vi "PSK.vi"() -> ()   [LabVIEW 2015]
panel:
  out "Waveform Graph":dbl[](graph)=[0.0, 0.9510565162951535, 0.5877852522924732, -0.5877852522924734, -0.9510565162951536, -2.4492935982947064e-16, 0.9510565162951538, 0.5877852522924734, -0.5877852522924728, -0.9510565162951538, -4.898587196589413e-16, 0.951056516295154, 0.5877852522924721, -0.5877852522924726, -0.9510565162951538, -7.347880794884119e-16, 0.9510565162951533, 0.5877852522924709, -0.5877852522924724, -0.9510565162951539, -9.797174393178826e-16, 0.9510565162951533, 0.5877852522924711, -0.5877852522924751, -0.9510565162951529, -1.2246467991473533e-15, -0.9510565162951532, -0.5877852522924742, 0.587785252292472, 0.9510565162951519, 1.4695761589768238e-15, -0.9510565162951531, -0.5877852522924744, 0.5877852522924718, 0.9510565162951519, 1.7145055188062944e-15, -0.951056516295153, -0.5877852522924746, 0.5877852522924716, 0.951056516295152, 1.959434878635765e-15, -0.9510565162951552, -0.5877852522924748, 0.5877852522924714, 0.9510565162951521, 2.204364238465236e-15, -0.9510565162951551, -0.587785252292475, 0.587785252292477, 0.9510565162951521, 2.4492935982947065e-15, 0.951056516295155, 0.5877852522924751, -0.5877852522924768, -0.9510565162951544, -9.799650315725178e-15, 0.9510565162951528, 0.5877852522924696, -0.5877852522924824, -0.9510565162951523, -2.9391523179536475e-15, 0.9510565162951549, 0.5877852522924756, -0.5877852522924764, -0.9510565162951545, 3.921345679817883e-15, 0.9510565162951525, 0.58778525229247, -0.5877852522924819, -0.9510565162951524, -3.429011037612589e-15, 0.9510565162951546, 0.587785252292476, -0.587785252292476, -0.9510565162951546, -1.0779367755043061e-14, -0.9510565162951524, -0.5877852522924705, 0.5877852522924816, 0.9510565162951525, 3.91886975727153e-15, -0.9510565162951502, -0.5877852522924649, 0.5877852522924756, 0.9510565162951549, -2.941628240500001e-15, -0.9510565162951523, -0.5877852522924708, 0.5877852522924811, 0.9510565162951528, 4.408728476930472e-15, -0.95105651629515, -0.5877852522924653, 0.5877852522924751, 0.951056516295155, 1.1759085194360944e-14, -0.9510565162951565, -0.5877852522924712, 0.5877852522924807, 0.9510565162951529, 4.898587196589413e-15, 0.9510565162951586, 0.5877852522924657, -0.5877852522924862, -0.9510565162951552, 1.9619108011821185e-15, 0.9510565162951563, 0.5877852522924601, -0.5877852522924688, -0.951056516295153, -1.9599300631450357e-14, 0.9510565162951585, 0.5877852522924776, -0.5877852522924744, -0.9510565162951509, -1.2738802633678827e-14, 0.9510565162951606, 0.587785252292472, -0.5877852522924799, -0.9510565162951575]
  out "Modulating wave 2":dbl[](graph)=[0.0, 0.9510565162951535, 0.5877852522924732, -0.5877852522924734, -0.9510565162951536, -2.4492935982947064e-16, 0.9510565162951538, 0.5877852522924734, -0.5877852522924728, -0.9510565162951538, -4.898587196589413e-16, 0.951056516295154, 0.5877852522924721, -0.5877852522924726, -0.9510565162951538, -7.347880794884119e-16, 0.9510565162951533, 0.5877852522924709, -0.5877852522924724, -0.9510565162951539, -9.797174393178826e-16, 0.9510565162951533, 0.5877852522924711, -0.5877852522924751, -0.9510565162951529, -1.2246467991473533e-15, 0.9510565162951532, 0.5877852522924742, -0.587785252292472, -0.9510565162951519, -1.4695761589768238e-15, 0.9510565162951531, 0.5877852522924744, -0.5877852522924718, -0.9510565162951519, -1.7145055188062944e-15, 0.951056516295153, 0.5877852522924746, -0.5877852522924716, -0.951056516295152, -1.959434878635765e-15, 0.9510565162951552, 0.5877852522924748, -0.5877852522924714, -0.9510565162951521, -2.204364238465236e-15, 0.9510565162951551, 0.587785252292475, -0.587785252292477, -0.9510565162951521, -2.4492935982947065e-15, 0.951056516295155, 0.5877852522924751, -0.5877852522924768, -0.9510565162951544, -9.799650315725178e-15, 0.9510565162951528, 0.5877852522924696, -0.5877852522924824, -0.9510565162951523, -2.9391523179536475e-15, 0.9510565162951549, 0.5877852522924756, -0.5877852522924764, -0.9510565162951545, 3.921345679817883e-15, 0.9510565162951525, 0.58778525229247, -0.5877852522924819, -0.9510565162951524, -3.429011037612589e-15, 0.9510565162951546, 0.587785252292476, -0.587785252292476, -0.9510565162951546, -1.0779367755043061e-14, 0.9510565162951524, 0.5877852522924705, -0.5877852522924816, -0.9510565162951525, -3.91886975727153e-15, 0.9510565162951502, 0.5877852522924649, -0.5877852522924756, -0.9510565162951549, 2.941628240500001e-15, 0.9510565162951523, 0.5877852522924708, -0.5877852522924811, -0.9510565162951528, -4.408728476930472e-15, 0.95105651629515, 0.5877852522924653, -0.5877852522924751, -0.951056516295155, -1.1759085194360944e-14, 0.9510565162951565, 0.5877852522924712, -0.5877852522924807, -0.9510565162951529, -4.898587196589413e-15, 0.9510565162951586, 0.5877852522924657, -0.5877852522924862, -0.9510565162951552, 1.9619108011821185e-15, 0.9510565162951563, 0.5877852522924601, -0.5877852522924688, -0.951056516295153, -1.9599300631450357e-14, 0.9510565162951585, 0.5877852522924776, -0.5877852522924744, -0.9510565162951509, -1.2738802633678827e-14, 0.9510565162951606, 0.587785252292472, -0.5877852522924799, -0.9510565162951575]
  out "Numeric 2":dbl=-3.4932993997482953e-16
  in  "phase 2":dbl
  in  "Amplitude 2":dbl=1.0
  in  "Fs 2":dbl=500.0
  in  "Frequency 2":dbl=100.0
  in  "No of Iteration 2":i32=120
  out "Modulating wave":dbl[](graph)=[0.0, 1.0, 1.0, 1.0, 1.0, 1.0, 1.0, 1.0, 1.0, 1.0, 1.0, 1.0, 1.0, 1.0, 1.0, 1.0, 1.0, 1.0, 1.0, 1.0, 1.0, 1.0, 1.0, 1.0, 1.0, 1.0, -1.0, -1.0, -1.0, -1.0, -1.0, -1.0, -1.0, -1.0, -1.0, -1.0, -1.0, -1.0, -1.0, -1.0, -1.0, -1.0, -1.0, -1.0, -1.0, -1.0, -1.0, -1.0, -1.0, -1.0, -1.0, 1.0, 1.0, 1.0, 1.0, 1.0, 1.0, 1.0, 1.0, 1.0, 1.0, 1.0, 1.0, 1.0, 1.0, 1.0, 1.0, 1.0, 1.0, 1.0, 1.0, 1.0, 1.0, 1.0, 1.0, 1.0, -1.0, -1.0, -1.0, -1.0, -1.0, -1.0, -1.0, -1.0, -1.0, -1.0, -1.0, -1.0, -1.0, -1.0, -1.0, -1.0, -1.0, -1.0, -1.0, -1.0, -1.0, -1.0, -1.0, -1.0, -1.0, 1.0, 1.0, 1.0, 1.0, 1.0, 1.0, 1.0, 1.0, 1.0, 1.0, 1.0, 1.0, 1.0, 1.0, 1.0, 1.0, 1.0, 1.0, 1.0]
  out "Numeric":dbl=0.014082858244057282
  in  "phase":dbl
  in  "Amplitude":dbl=1.0
  in  "Fs":dbl=1000.0
  in  "Frequency":dbl=20.0
  in  "No of Iteration":i32=120
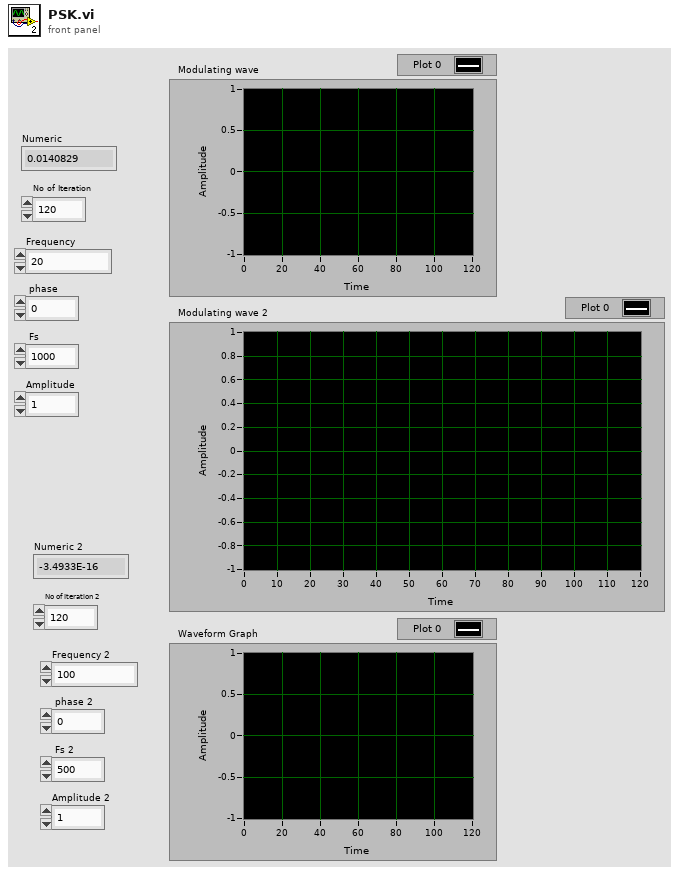
[diagram p1: front panel]
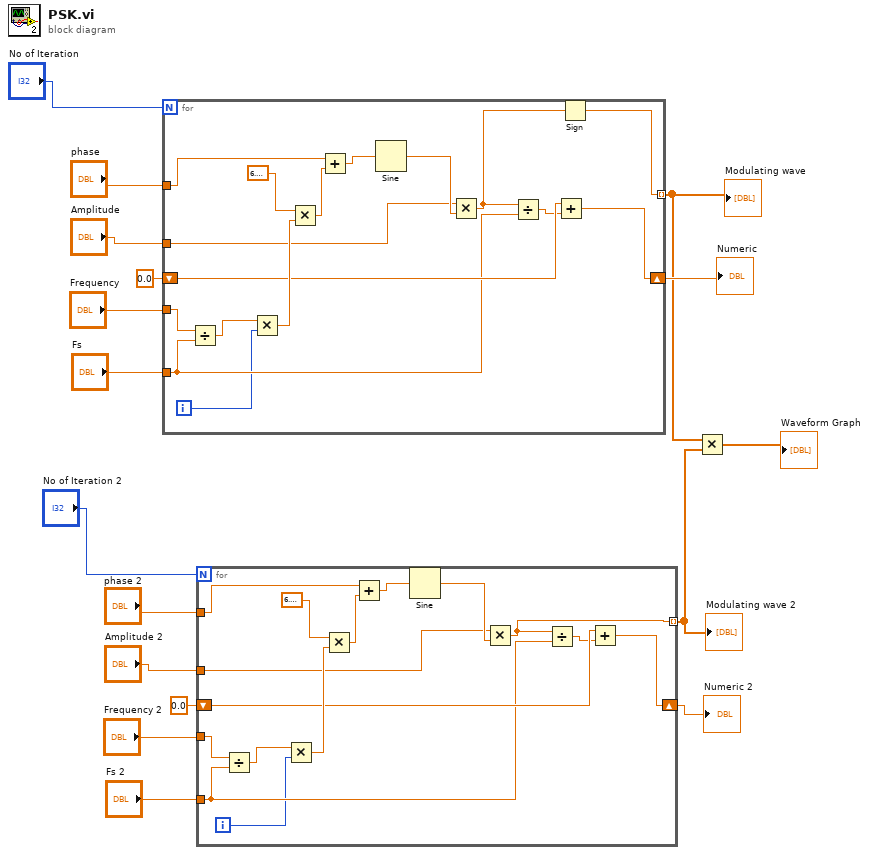
[diagram p0: block diagram]
diagram:
  n1 = for {
    N: "No of Iteration" -> [_]
    tunnel: "Frequency" -> [w32]
    tunnel: "Fs" -> [w22]
    tunnel: "Amplitude" -> [w28]
    tunnel: "phase" -> [w27]
    shift-right: [w20] -> w12
    shift-left: 0.0 -> [w25]
    tunnel: [w19] -> w2 mode=indexing
    i -> [w21]
    n2 = Divide(x=w32, y=w22) -> (x/y=w26:dbl)
    n3 = Multiply(x=w26, y=w21) -> (x*y=w30:dbl)
    n4 = Multiply(x=6.283185307179586, y=w30) -> (x*y=w31:dbl)
    n5 = Add(x=w27, y=w31) -> (x+y=w33:dbl)
    n6 = Sine(x=w33) -> (sin(x)=w29:dbl)
    n7 = Multiply(x=w28, y=w29) -> (x*y=w18:dbl)
    n8 = Divide(x=w18, y=w22) -> (x/y=w23:dbl)
    n9 = Add(x=w25, y=w23) -> (x+y=w20:dbl)
    n10 = Sign(1:w18) -> (0:w19:dbl)
  }
  "Numeric" <- w12
  "Modulating wave" <- w2
  n11 = for {
    N: "No of Iteration 2" -> [_]
    tunnel: "Frequency 2" -> [w47]
    tunnel: "Fs 2" -> [w37]
    tunnel: "Amplitude 2" -> [w43]
    tunnel: "phase 2" -> [w42]
    shift-right: [w35] -> w5
    shift-left: 0.0 -> [w40]
    tunnel: [w34] -> w3 mode=indexing
    i -> [w36]
    n12 = Divide(x=w47, y=w37) -> (x/y=w41:dbl)
    n13 = Multiply(x=w41, y=w36) -> (x*y=w45:dbl)
    n14 = Multiply(x=6.283185307179586, y=w45) -> (x*y=w46:dbl)
    n15 = Add(x=w42, y=w46) -> (x+y=w48:dbl)
    n16 = Sine(x=w48) -> (sin(x)=w44:dbl)
    n17 = Multiply(x=w43, y=w44) -> (x*y=w34:dbl)
    n18 = Divide(x=w34, y=w37) -> (x/y=w38:dbl)
    n19 = Add(x=w40, y=w38) -> (x+y=w35:dbl)
  }
  "Numeric 2" <- w5
  "Modulating wave 2" <- w3
  n20 = Multiply(x=w2, y=w3) -> (x*y=→"Waveform Graph":dbl[])
